vi "Append Pass Result.vi"(7 "Description":string, 8 "error in (no error)":errorcluster, 9 "Message":string, 10 "Result Type":T1, 11 "LUnit Test Case In":refnum<class "LUnit Test Case.lvclass">) -> (0 "error out":errorcluster, 3 "LUnit Test Case Out":refnum<class "LUnit Test Case.lvclass">)   [LabVIEW 2020, in "LUnit Test Case.lvclass"]
doc: "Generates a pass result for the calling test method. A description and message may be provided."
uses:
  LUnit Test Case.lvclass
  Core/Result/Type.ctl
  Core/Result/Result.ctl
  Core/Result/Status.ctl
  LUnit Test Case.lvclass/LUnit Test Case.ctl
  Core/Result/Result.lvlib
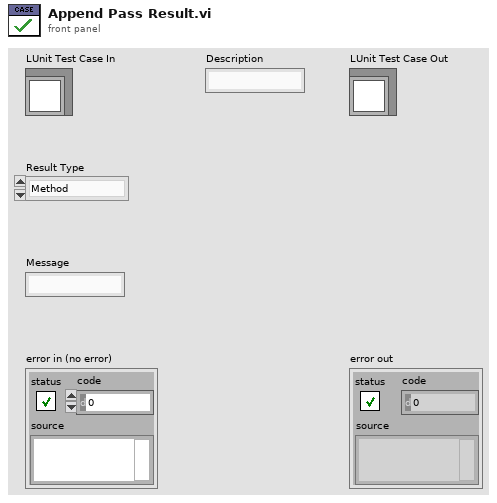
[diagram p1: front panel]
types:
  T1 = typedef "Result.lvlib/Type.ctl" = enum16{"Method", "Case", "Suite", "Pass", "Fail", "Skip", "Pass if", "Fail if", "Pass if Error", "Fail if Error", "Pass if Equal", "Fail if Equal"}
  T2 = typedef "Result.lvlib/Result.ctl" = cluster{"Name":string, "Message":string, "Description":string, "Status":T3, "Result Type":T1, "Execution Time":dbl}
  T3 = typedef "Result.lvlib/Status.ctl" = enum16{"", "Passed", "Failed", "Error", "Skipped", "Setup Error", "Broken", "Teardown Error"}
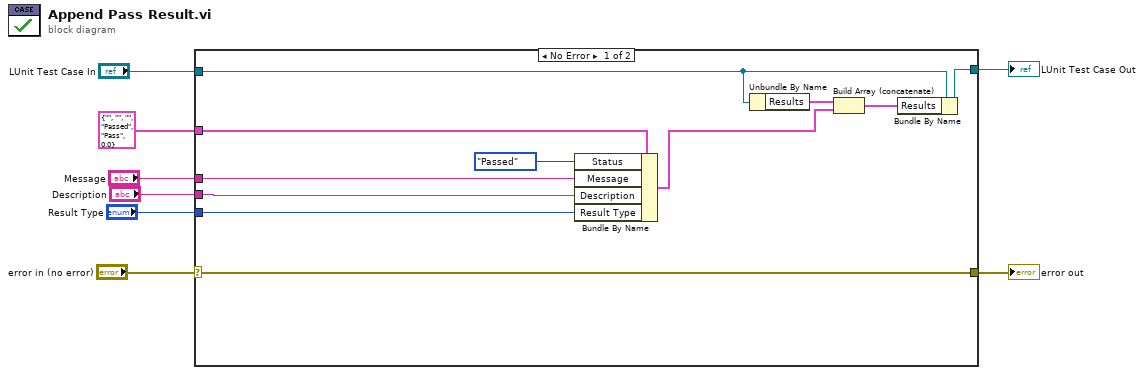
[diagram p0: block diagram]
diagram:
  n1 = case shown="No Error" "error in (no error)" {
    selector: "error in (no error)" -> [w18 w20]
    tunnel: "LUnit Test Case In" -> [w19 w21]
    tunnel: [w18 w20] -> w6
    tunnel: "Message" -> [w17 _]
    tunnel: "Description" -> [w16 _]
    tunnel: T2 {"Name"="", "Message"="", "Description"="", "Status"=enum."Passed", "Result Type"=enum."Pass", "Execution Time"=0.0} ("Temporary Assertion Result") -> [w15 _]
    tunnel: [w14 w21] -> w2
    tunnel: "Result Type" -> [w12 _]
    frame No Error {
      n2 = Bundle By Name(cluster=w15, "Status"=Status."Passed", "Message"=w17, "Description"=w16, "Result Type"=w12) -> (w13:T2)
      n3 = Unbundle By Name(w19) -> ("Results"=w11:T2[])
      n4 = Build Array (concatenate)(w11, w13) -> (w10:T2[])
      n5 = Bundle By Name(cluster=w19, "Results"=w10) -> (w14:refnum<class "LUnit Test Case.lvclass">)
    }
    frame Error {
    }
  }
  "error out" <- w6
  "LUnit Test Case Out" <- w2
